vi "Set RFFE Adress.vi"(8 "error in (no error)":errorcluster, 10 "Physical Adress":u32, 11 "VISA resource name":refnum<visa-resource-name>) -> (0 "error out":errorcluster, 3 "VISA resource name out":refnum<visa-resource-name>)   [LabVIEW 2020, in "PIC-Device.lvclass"]
doc: "Setting the RFFE Physical adress"
uses:
  PIC-Device.lvclass
  <vilib>/Instr/_visa.llb/Select Event Type.ctl
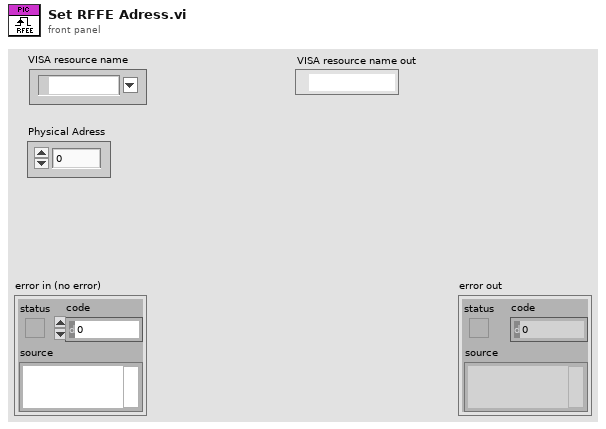
[diagram p1: front panel]
types:
  T1 = typedef "Select Event Type.ctl" = u32
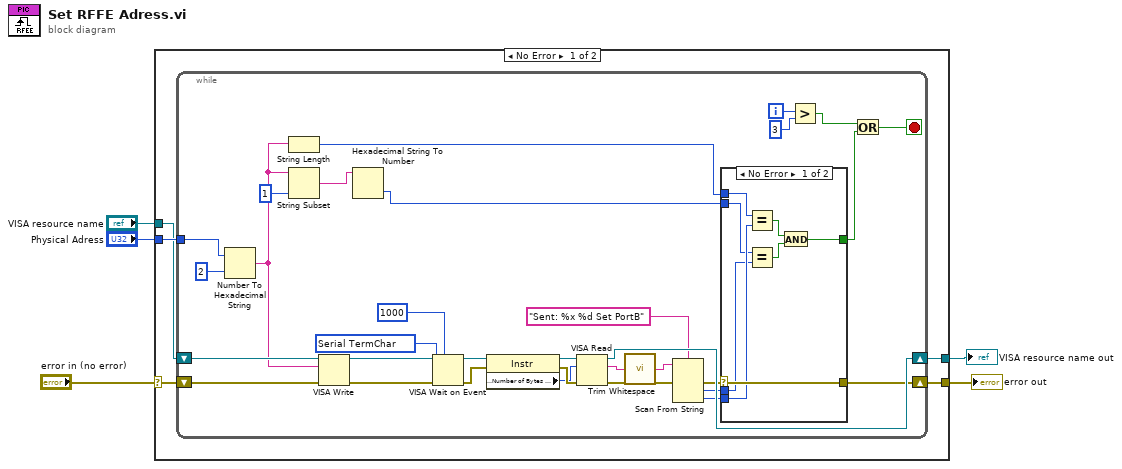
[diagram p0: block diagram]
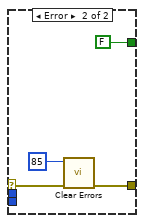
[diagram p2: hidden frame]
diagram:
  n1 = case shown="No Error" "error in (no error)" {
    selector: "error in (no error)" -> [w10 w56]
    tunnel: [w6 w56] -> w4
    tunnel: "VISA resource name" -> [w8 w55]
    tunnel: "Physical Adress" -> [w9 _]
    tunnel: [w7 w55] -> w1
    frame No Error {
      n2 = while {
        tunnel: w9 -> [w41]
        shift-right: [w25] -> w7
        shift-left: w8 -> [w39]
        shift-right: [w14] -> w6
        shift-left: w10 -> [w42]
        i -> [w13]
        stop <- w15 stop-if-true
        w32 = T1 1073684516 items=["Service Request"=1073684491, "Trigger"=3221168138, "Clear"=1073684493, "VXI Signal"=1073684512, "VXI/VME Interrupt"=3221168161, "VXI/VME Sysfail"=1073684509, "VXI/VME Sysreset"=1073684510, "GPIB CIC"=1073684498, "GPIB Talk"=1073684499, "GPIB Listen"=1073684500, "PXI Interrupt"=1073684514, "Serial Break"=1073684515, "Serial TermChar"=1073684516, "Serial CTS"=1073684521, "Serial DSR"=1073684522, "Serial DCD"=1073684524, "Serial RI"=1073684526, "Serial Character"=1073684533, "USB Interrupt"=1073684535, "All Enabled"=1073709055] ("Event Type")
        n3 = Number To Hexadecimal String(1:i16 2 ("width (-)"), 2:w41) -> (0:w38:string)
        n4 = String Length(string=w38) -> (length=w18:i32)
        n5 = String Subset(string=w38, length (rest)=1 ("length (rest)")) -> (substring=w36:string)  [unwired: 1 in]
        n6 = VISA Write(VISA resource name=w39, write buffer=w38, error in (no error)=w42) -> (VISA resource name out=w34:refnum<visa-resource-name>, error out=w35:errorcluster)  [unwired: 1 out]
        n7 = Hexadecimal String To Number(string=w36) -> (number=w17:u32)  [unwired: 2 in, 1 out]
        n8 = VISA Wait on Event(7:u32 1000 ("timeout (0)"), 8:w35, 10:w32, 11:w34) -> (0:w30:errorcluster, 3:w31:refnum<visa-resource-name>)  [unwired: 1 in, 2 out]
        n9 = property class="Instr"(reference=w31, error in=w30) -> (reference out=w27:refnum<visa-resource-name>, error out=w29:errorcluster, "Serial Settings:Number of Bytes at Serial Port"=w28:u32)
        n10 = VISA Read(VISA resource name=w27, byte count=w28, error in (no error)=w29) -> (VISA resource name out=w25:refnum<visa-resource-name>, read buffer=w26:string, error out=w23:errorcluster)  [unwired: 1 out]
        n11 = call <vilib>:"Trim Whitespace.vi"("string"=w26) -> ("trimmed string"=w24:string)  [unwired: 1 in]
        n12 = Scan From String(format string="Sent: %x %d Set PortB", input string=w24, error in=w23) -> (error out=w21:errorcluster, output 1=w20:u32, output 2=w19:i32)  [unwired: 3 in, 2 out]
        n13 = case shown="No Error" w21 {
          selector: w21 -> [w50 w53]
          tunnel: [w50 w54] -> w14
          tunnel: w20 -> [w47 _]
          tunnel: w19 -> [w48 _]
          tunnel: w18 -> [w49 _]
          tunnel: w17 -> [w46 _]
          tunnel: [w43 FALSE] -> w16
          frame No Error {
            n14 = Equal?(x=w49, y=w48) -> (x = y?=w44:bool)
            n15 = Equal?(x=w46, y=w47) -> (x = y?=w45:bool)
            n16 = And(x=w44, y=w45) -> (x .and. y?=w43:bool)
          }
          frame Error {
            n17 = call <vilib>:"Clear Errors.vi"("error in (no error)"=w53, "specific error code to clear (0: all)"=85) -> ("error out"=w54:errorcluster)  [unwired: 4 in, 1 out]
          }
        }
        n18 = Greater?(x=w13, y=3) -> (0:w11:bool)
        n19 = Or(x=w11, y=w16) -> (x .or. y?=w15:bool)
      }
    }
    frame Error {
    }
  }
  "error out" <- w4
  "VISA resource name out" <- w1
